vi "findAllPollers.vi"(11 "ttm_poller_panel_in":refnum<class "ttmServer.lvclass">) -> (2 "pollerFileNames":string[](array[string]), 3 "ttm_poller_panel_out":refnum<class "ttmServer.lvclass">)   [LabVIEW 2011, in "ttmServer.lvclass"]
uses:
  ttmServer.lvclass
  ttmServer.lvclass/ttmServer.ctl
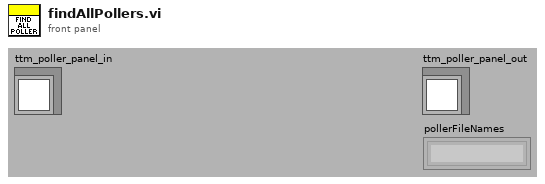
[diagram p1: front panel]
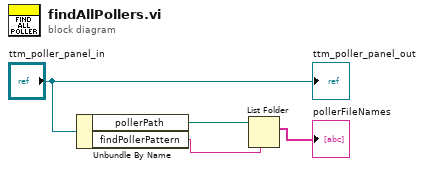
[diagram p0: block diagram]
diagram:
  n1 = Unbundle By Name("ttm_poller_panel_in") -> ("pollerPath"=w3:path, "findPollerPattern"=w2:string)
  n2 = List Folder(path=w3, pattern=w2) -> (filenames=→"pollerFileNames":string[])  [unwired: 2 in, 3 out]
  "ttm_poller_panel_out" <- "ttm_poller_panel_in"
